vi "set_voltage_and_current.vi"(8 "error in":errorcluster, 9 "current":dbl, 10 "voltage":dbl, 11 "VISA resource name":refnum<visa-resource-name>="COM1") -> (0 "error out":errorcluster, 2 "command":string, 3 "Response":string)   [LabVIEW 2020]
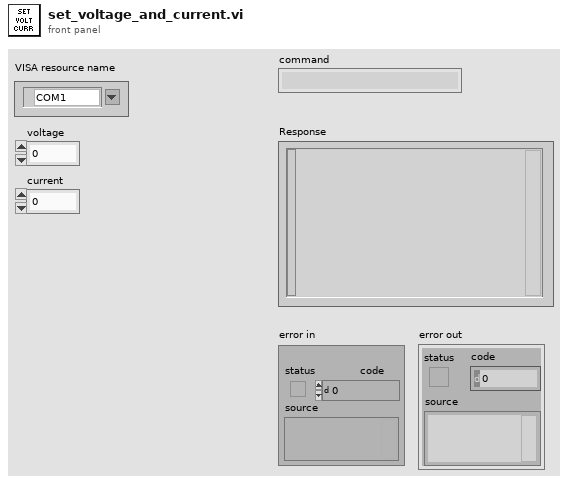
[diagram p1: front panel]
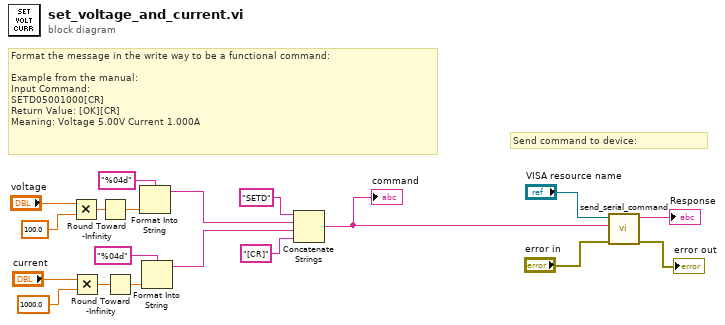
[diagram p0: block diagram]
diagram:
  # "Send command to device:"
  # "Format the message in the write way to be a functional command:\n\nExample from the manual:\nInput Command:\nSETD05001000[CR]\nReturn Value: [OK][CR]\nMeaning: Voltage 5.00V Current 1.000A"
  n1 = Multiply(x="voltage", y=100.0) -> (x*y=w13:dbl)
  n2 = Multiply(x="current", y=1000.0) -> (x*y=w12:dbl)
  n3 = Round Toward -Infinity(1:w13) -> (0:w9:dbl)
  n4 = Round Toward -Infinity(1:w12) -> (0:w7:dbl)
  n5 = Format Into String(format string="%04d", w9) -> (resulting string=w10:string)  [unwired: 2 in, 1 out]
  n6 = Format Into String(format string="%04d", w7) -> (resulting string=w6:string)  [unwired: 2 in, 1 out]
  n7 = Concatenate Strings("SETD" ("string"), w10, w6, "[CR]" ("string")) -> (w1:string)
  "command" <- w1
  n8 = call "send_serial_command.vi"("error in (no error)"="error in", "Command"=w1, "VISA resource name"="VISA resource name") -> ("error out"=→"error out":errorcluster, "Response"=→"Response":string)  [unwired: 7 in]
